vi "Autonomous Independent.vi"() -> ()   [LabVIEW 2014]
doc: "This VI is called when autonomous begins, and will automatically be terminated when autonomous ends. You can carry out timed or sensor driven robot movement independently without needing to return to the caller."
uses:
  Auto/Autonomous Modes.ctl
  Elevator/Elevator States.ctl
  Arms/Arm clapper state.ctl
  Utilities/Sensor Refname.ctl
  Utilities/Sensor Refname to String.vi
  <vilib>/Rock Robotics/Network Tables/SD Read Number.vi
panel:
  in  "Turn gyro":T1={"proportional gain (Kc)"=-0.05625, "integral time (Ti, min)"=0.0, "derivative time (Td, min)"=0.0} {"derivative time (Td, min)" format="%.3f"; "integral time (Ti, min)" format="%.3f"; "proportional gain (Kc)" format="%.3f"}
  in  "Third Forward Speed":dbl=0.7
  in  "Deposit Stack Drive Speed":dbl=-0.8 format="%#_13g"
  in  "Forward Speed Second Movement":dbl=0.65
  in  "Forward Speed into Zone":dbl=-0.8
  in  "Forward Speed First":dbl=0.8 format="%#_13g"
  in  "Distance (in)":dbl=57.0
  in  "Turn Left Distance (in)":dbl=90.0 format="%#_13g"
  in  "Turn Left Speed":dbl=0.75
  in  "Turn Right Speed":dbl=0.75
  in  "Turn Right Distance (in)":dbl=90.0 format="%#_13g"
  in  "Move Speed":dbl=0.75 format="%#_13g"
  in  "Move Time (s)":dbl=2.5 format="%#_13g"
  # "THREE TOTE"
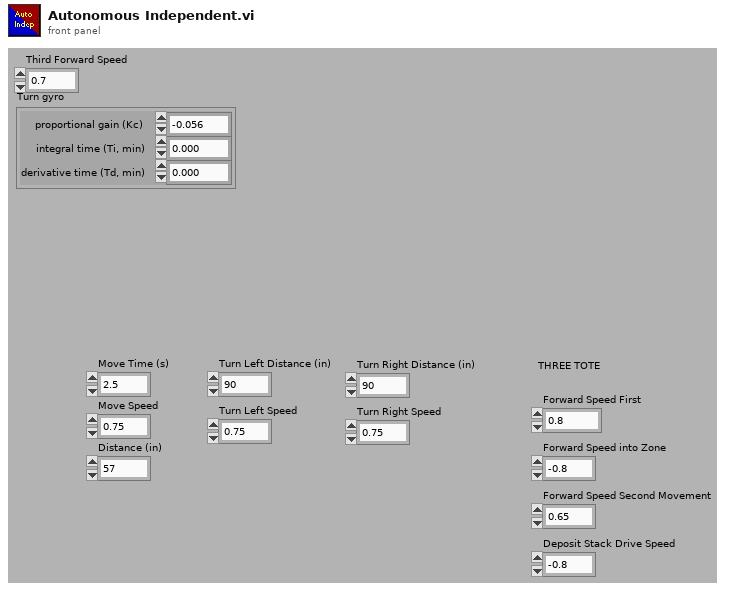
[diagram p1: front panel]
types:
  T1 = cluster{"proportional gain (Kc)":dbl, "integral time (Ti, min)":dbl, "derivative time (Td, min)":dbl}
  T2 = typedef "Autonomous Modes.ctl" = enum16{"3 Tote", "Turn Left, Drive to Auto", "Turn Right, Drive to Auto", "1 Bin", "Move To Auto Zone", "Do Nothing"}
  T3 = typedef "Auto Notifiers.ctl" = cluster{"Auto to Clap":refnum<notifier>, "Clap to Auto":refnum<notifier>, "Auto to Angle":refnum<notifier>, "Angle to Auto":refnum<notifier>, "Auto to Roller":refnum<notifier>, "Drive Distance Speed":refnum<notifier>, "Drive Distance Distance":refnum<notifier>, "Auto Done?":refnum<notifier>, "Keep Straight?":refnum<notifier>, "Turn 90?":refnum<notifier>}
  T4 = typedef "Auto Refs.ctl" = cluster{"Ultrasonic Forward":T5, "Ultrasonic Back":T5, "Strafe Motor":T9, "Drive Motors":T18, "Gyro":T19}
  T5 = typedef "WPI_SonarMB1010AnalogDeviceRef.ctl" = cluster{"AIDeviceRef":T6, "Scaling factor (V/in)":dbl, "Average Bits":u8}
  T6 = typedef "WPI_AnalogChannelDevRef.ctl" = cluster{"DevStatus":errorcluster, "Controller":T7, "Analog Channel":T8}
  T7 = typedef "FPGA_TypedefAnalogModule.ctl" = enum16{"Controller 1"}
  T8 = typedef "FPGA_AIChannel.ctl" = enum8{"AI 0", "AI 1", "AI 2", "AI 3", "AI MXP 0", "AI MXP 1", "AI MXP 2", "AI MXP 3", "Invalid"}
  T9 = typedef "WPI_MotorControlDeviceRef.ctl" = cluster{"DeviceStatus":errorcluster, "Type":T10, "PWM":cluster{"Controller":T11, "PWM Channel":T12, "DeadBand":T13}, "CAN":cluster{"Device Number":u8, "Control Mode":T14, "Semaphore":T15, "Max Vout":dbl, "TalonSRX Control Mode":T16}, "Invert":bool, "TransformRef":T17, "InvTransformRef":T17}
  T10 = typedef "WPI_MotorControlType.ctl" = enum16{"PWM", "CAN", "CANTalonSRX"}
  T11 = typedef "FPGA_TypedefDigitalModule.ctl" = enum16{"Controller 1"}
  T12 = typedef "FPGA_DIOPWMChannel.ctl" = enum8{"PWM 0", "PWM 1", "PWM 2", "PWM 3", "PWM 4", "PWM 5", "PWM 6", "PWM 7", "PWM 8", "PWM 9", "PWM MXP 0", "PWM MXP 1", "PWM MXP 2", "PWM MXP 3", "PWM MXP 4", "PWM MXP 5", "PWM MXP 6", "PWM MXP 7", "PWM MXP 8", "PWM MXP 9", "Invalid"}
  T13 = typedef "WPI_PWMDeadband.ctl" = cluster{"Name":string, "maxPositivePwm":i32, "minPositivePwm":i32, "centerPwm":i32, "maxNegativePwm":i32, "minNegativePwm":i32, "angularRange":u16}
  T14 = typedef "WPI_CANJaguar_ControlMode.ctl" = enum8{"Percent VBus", "Current", "Speed", "Position", "Voltage"}
  T15 = typedef "Semaphore RefNum" = refnum<k1>
  T16 = typedef "WPI_CANTalonSRX_APIControlMode.ctl" = enum8{"Percent VBus", "Speed", "Position", "Slave", "Unchanged / Invalid"}
  T17 = typedef "WPI_PWMTransform_ConPane.ctl" = refnum<vi>
  T18 = typedef "WPI_RobotDriveDevRef.ctl" = cluster{"DevStatus":errorcluster, "Motors[]":T9[], "Square Inputs":bool, "Max Output":dbl}
  T19 = typedef "WPI_GyroDevRef.ctl" = cluster{"DevStatus":errorcluster, "Analog Module":T7, "Analog Channel":T8, "Offset":dbl, "Gain (VoltsPerDegree/Second)":dbl}
  T20 = typedef "Sensor Refname.ctl" = enum16{"Gyro", "Elevator Top LS", "Elevator Bottom LS", "Claw Outside LS", "Left Drive Encoder", "Right Drive Encoder", "Strafe Encoder", "Elevator Encoder", "Ultrasonic Forward", "Ultrasonic Back", "Arm Angle POT", "Arm Clapper POT", "Accelerometer", "Tote LS", "DIP 1", "DIP 2", "DIP 3", "DIP 4"}
  T21 = typedef "Arm clapper state.ctl" = enum16{"In", "Tote Closed", "Bin Closed", "Straight", "Open"}
  T22 = typedef "Elevator States.ctl" = enum16{"Ground", "Tote 1", "Tote 2", "Tote 3", "Tote 4", "Tote 5", "Tote 6"}
  T23 = typedef "WPI_SwitchDevRef.ctl" = cluster{"DevStatus":errorcluster, "DIO Channel":T24, "Controller":T11, "CntIndex":T25, "Normally Closed":bool}
  T24 = typedef "FPGA_DIOChannel.ctl" = enum8{"DIO 0", "DIO 1", "DIO 2", "DIO 3", "DIO 4", "DIO 5", "DIO 6", "DIO 7", "DIO 8", "DIO 9", "DIO MXP 0", "DIO MXP 1", "DIO MXP 2", "DIO MXP 3", "DIO MXP 4", "DIO MXP 5", "DIO MXP 6", "DIO MXP 7", "DIO MXP 8", "DIO MXP 9", "DIO MXP 10", "DIO MXP 11", "DIO MXP 12", "DIO MXP 13", "DIO MXP 14", "DIO MXP 15", "Invalid"}
  T25 = typedef "FPGA_CounterCtrSystemIndex.ctl" = enum8{"Ctr 0", "Ctr 1", "Ctr 2", "Ctr 3", "Ctr 4", "Ctr 5", "Ctr 6", "Ctr 7", "Invalid"}
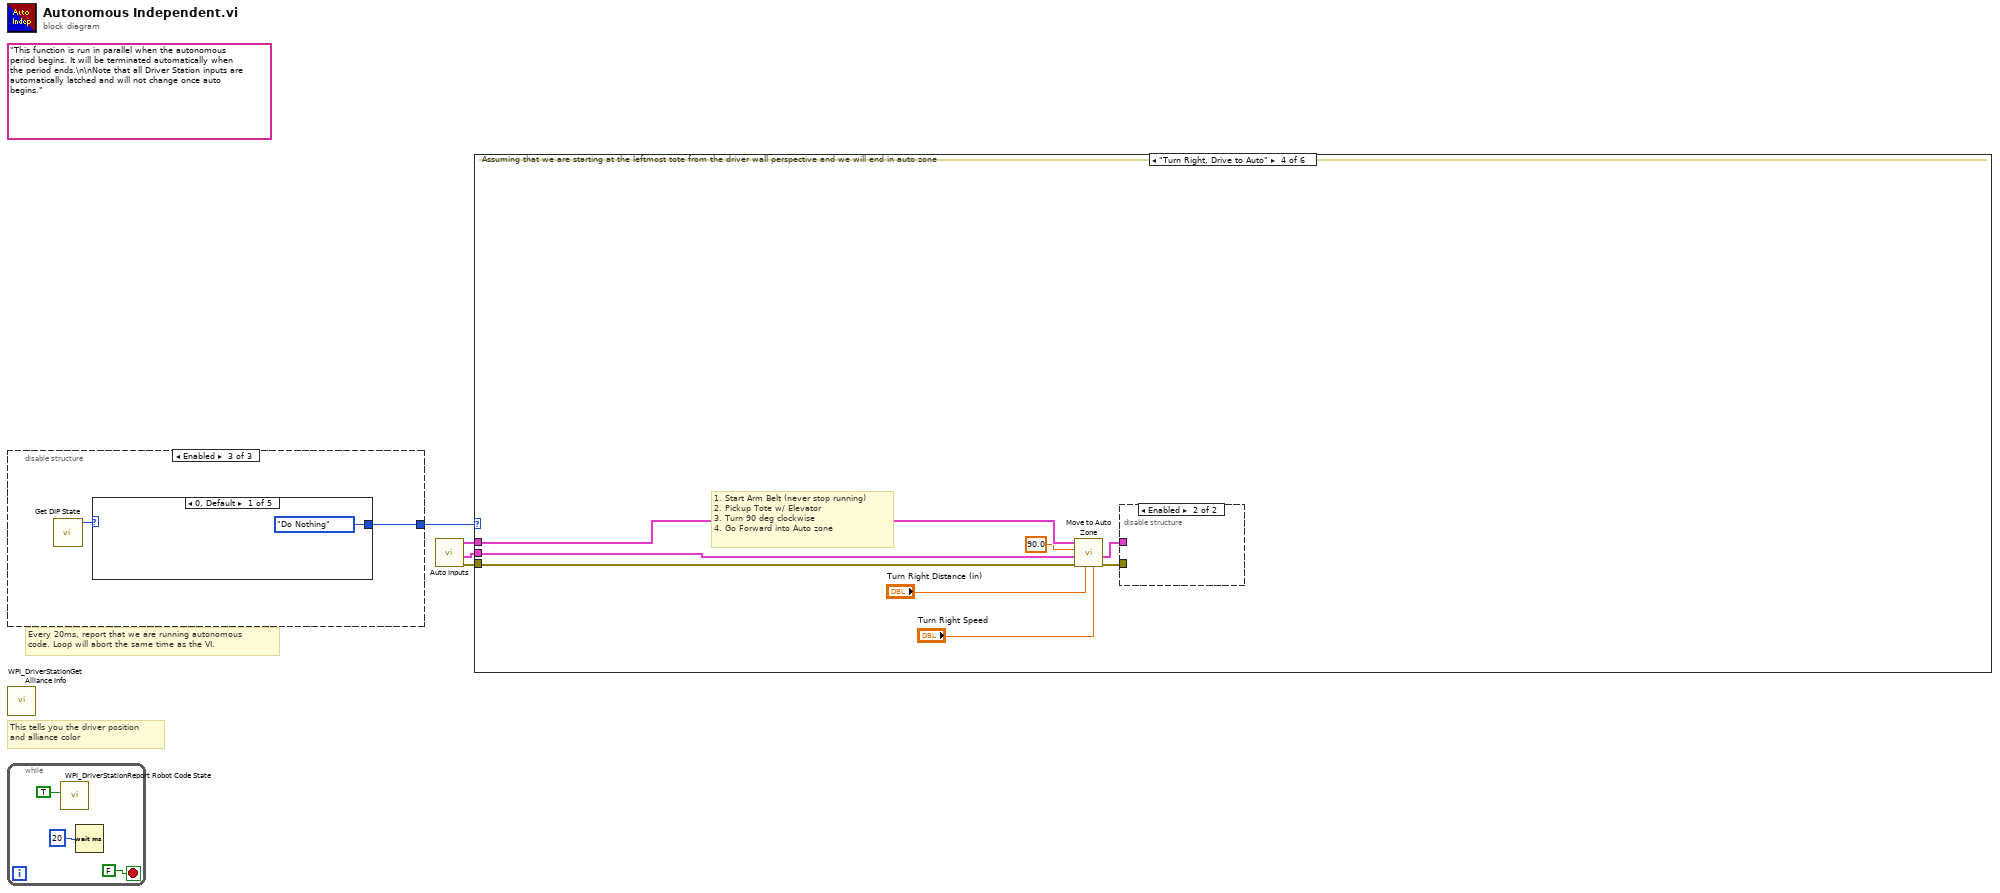
[diagram p0: block diagram]
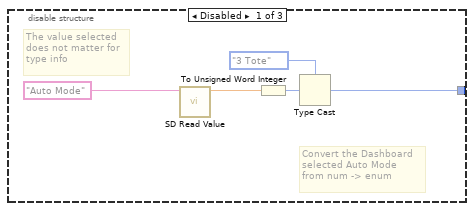
[diagram p2: hidden frame]
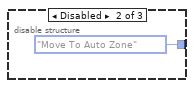
[diagram p3: hidden frame]
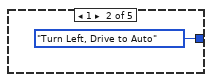
[diagram p4: hidden frame]
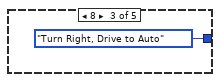
[diagram p5: hidden frame]
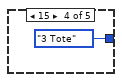
[diagram p6: hidden frame]
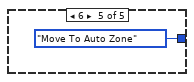
[diagram p7: hidden frame]
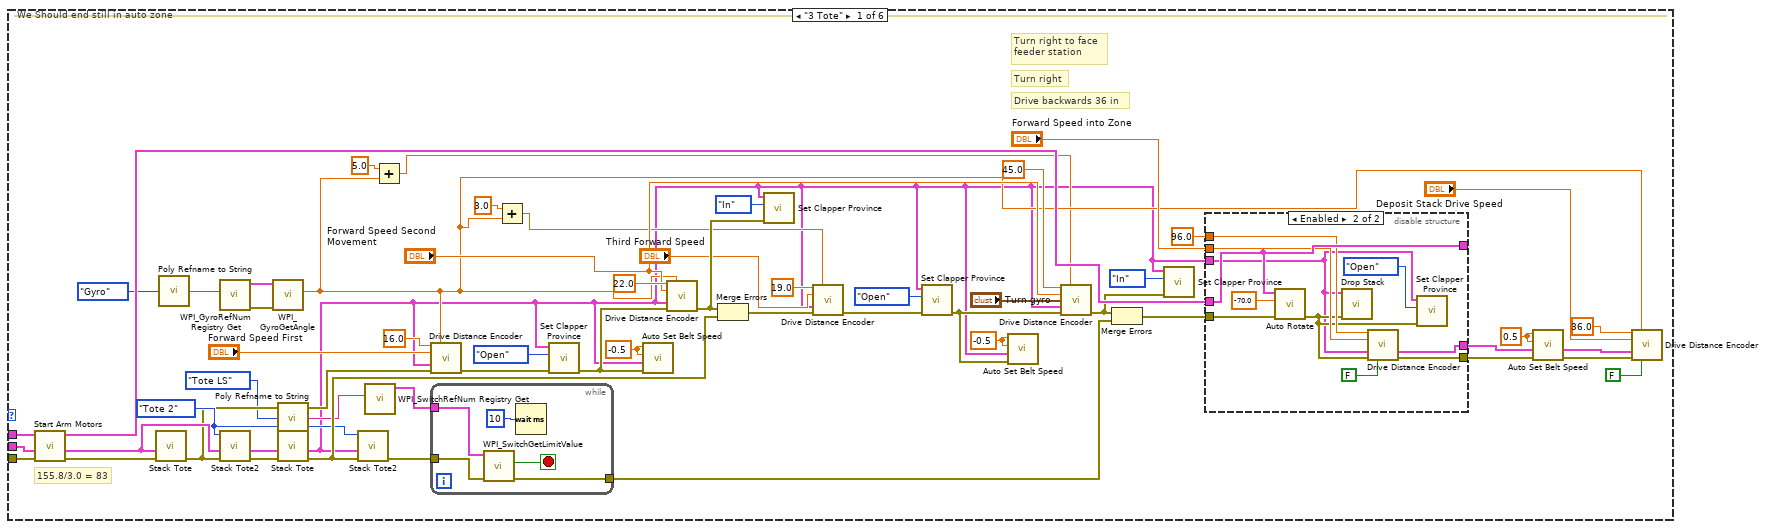
[diagram p8: hidden frame]
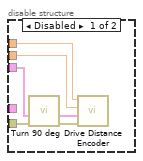
[diagram p9: hidden frame]
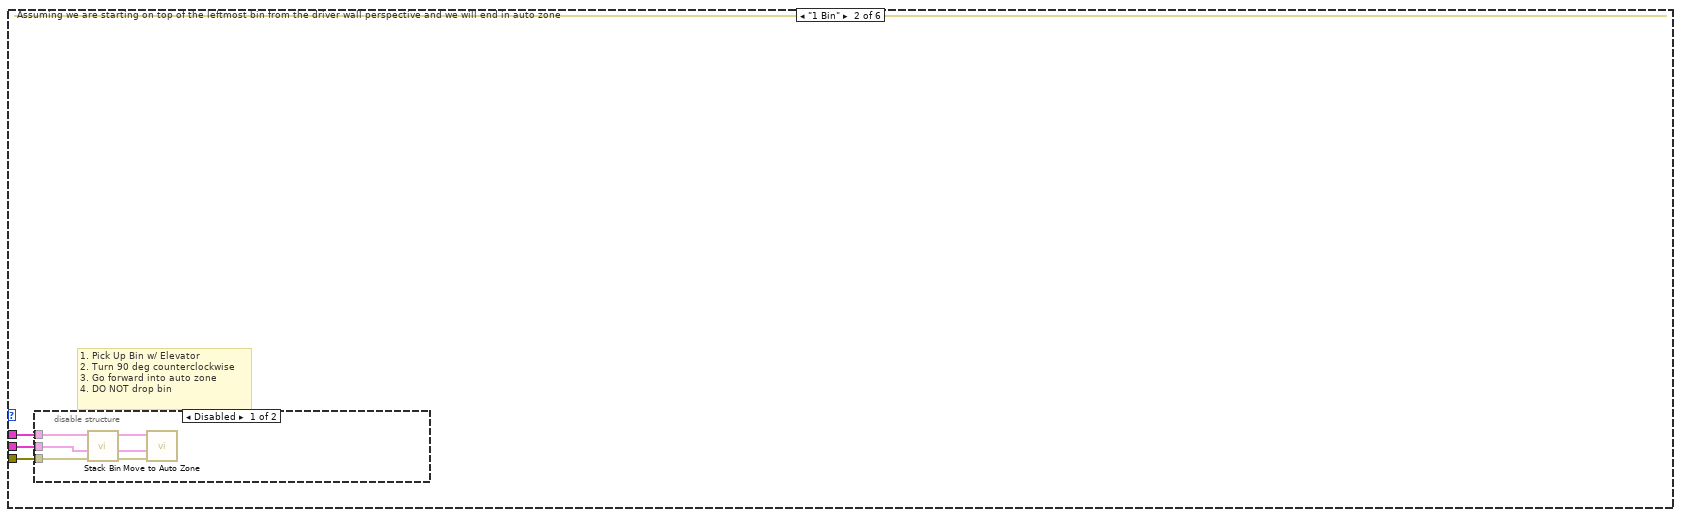
[diagram p10: hidden frame]
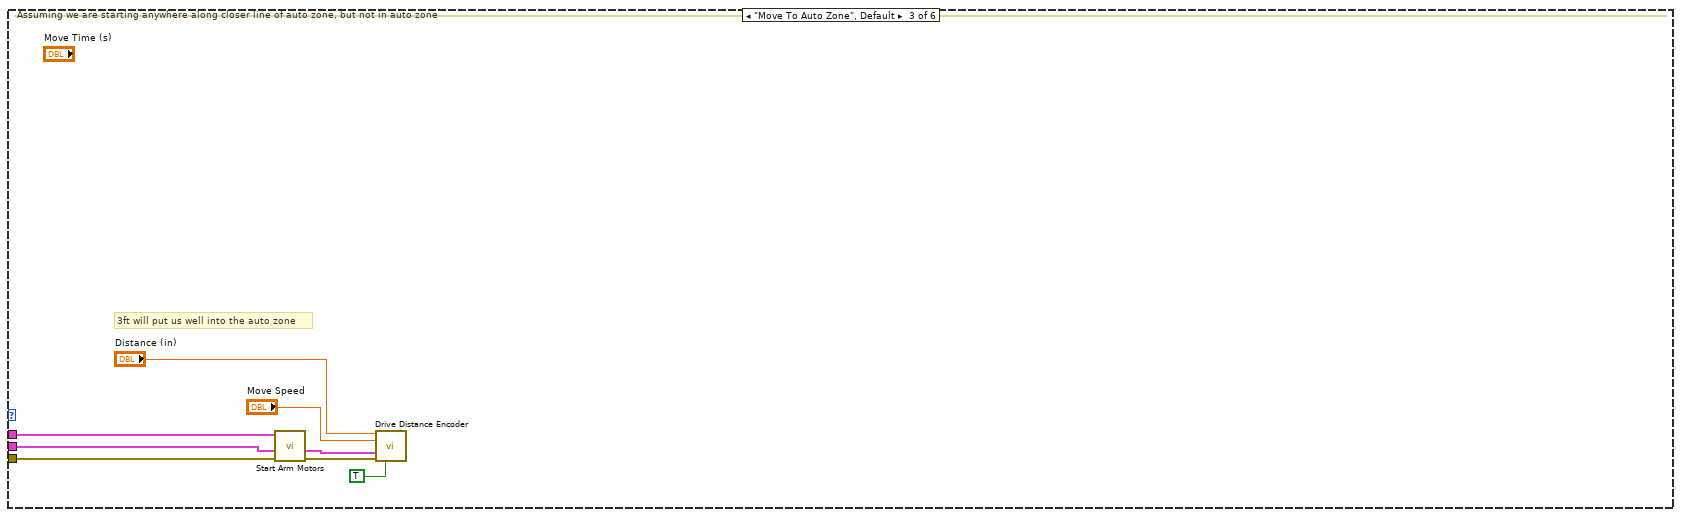
[diagram p12: hidden frame]
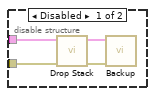
[diagram p13: hidden frame]
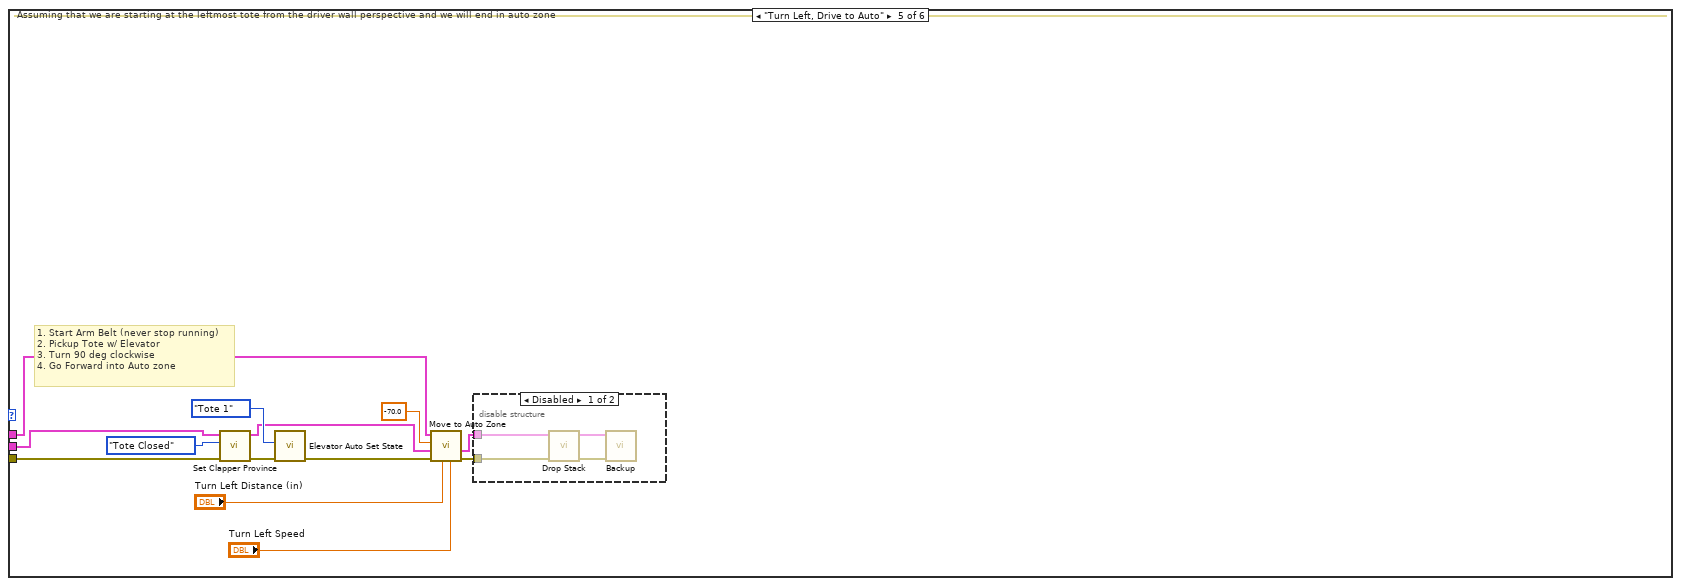
[diagram p14: hidden frame]
diagram:
  (unwired) "This function is run in parallel when the autonomous period begins. It will be terminated automatically when the period ends.\n\nNote that all Driver Station inputs are automatically latched and will not change once auto begins."
  # "Every 20ms, report that we are running autonomous\ncode. Loop will abort the same time as the VI."
  # "This tells you the driver position\nand alliance color"
  n1 = disable-structure shown="Enabled" {
    disable-tunnel: [w5 Autonomous_Modes."Move To Auto Zone" ("Auto Mode") w11] -> w1
    frame Disabled {
      # "The value selected\ndoes not matter for\ntype info"
      # "Convert the Dashboard\nselected Auto Mode\nfrom num -> enum"
      n2 = call-poly <vilib>:"SD Read Value.vi"("Name"="Auto Mode") -> ("Numeric"=w9:dbl)  [unwired: 8 in, 2 out]
      n3 = To Unsigned Word Integer(number=w9) -> (unsigned 16bit integer=w8:u16)
      n4 = Type Cast(type=Autonomous_Modes."3 Tote" ("Auto Mode"), x=w8) -> (*(type *) &x=w5:T2)
    }
    frame Disabled {
    }
    frame Enabled {
      n5 = call "Get DIP State.vi"() -> ("DIP State"=w12:u32)  [unwired: 10 in, 1 out]
      n6 = case shown="0, Default" w12 {
        tunnel: [Autonomous_Modes."Do Nothing" ("Auto Mode") Autonomous_Modes."Turn Left, Drive to Auto" ("Auto Mode") Autonomous_Modes."Turn Right, Drive to Auto" ("Auto Mode") Autonomous_Modes."3 Tote" ("Auto Mode") Autonomous_Modes."Move To Auto Zone" ("Auto Mode")] -> w11
        frame 0, Default {
        }
        frame 1 {
        }
        frame 8 {
        }
        frame 15 {
        }
        frame 6 {
        }
      }
    }
  }
  n7 = call <vilib>:"WPI_DriverStationGet Alliance Info.vi"() -> ()  [unwired: 12 out]
  n8 = while {
    stop <- FALSE stop-if-true
    n9 = call <vilib>:"WPI_DriverStationReport Robot Code State.vi"("Autonomous"=TRUE) -> ()  [unwired: 10 in, 1 out]
    n10 = Wait (ms)(milliseconds to wait=u32 20) -> ()  [unwired: 1 out]
  }
  n11 = call "Auto Inputs.vi"() -> ("error out"=w2:errorcluster, "Auto Notifiers Out"=w3:T3, "Auto Refs"=w4:T4)  [unwired: 9 in]
  n12 = case shown="\"Turn Right, Drive to Auto\"" w1 {
    tunnel: w4 -> [w76 w103 w112 w121 w139 _]
    tunnel: w3 -> [w78 w102 w114 w123 w133 _]
    tunnel: w2 -> [w77 w101 w116 w124 w141 _]
    frame "3 Tote" {
      w57 = -0.5 ("Right Belt")
      w68 = -0.5 ("Right Belt")
      w42 = Elevator_States."Tote 2" ("New State")
      w72 = 0.5
      # "Drive backwards 36 in"
      # "Turn right to face\nfeeder station"
      # "Turn right"
      # "155.8/3.0 = 83"
      # "We Should end still in auto zone"
      n13 = call "Start Arm Motors.vi"("error in"=w77, "Auto Notifiers In"=w78, "Auto Refs"=w76) -> ("error out"=w47:errorcluster, "Auto Notifiers Out"=w41:T3, "Auto Refs"=w74:T4)  [unwired: 6 in]
      n14 = call "Stack Tote.vi"("error in"=w47, "Auto Notifiers In"=w41) -> ("error out(no error)"=w38:errorcluster)  [unwired: 8 in, 1 out]
      n15 = call-poly "Poly Refname to String.vi"("Sensor Refnames"=Sensor_Refname."Gyro") -> ("Refname"=w49:string)
      n16 = call <vilib>:"WPI_GyroRefNum Registry Get.vi"("refnum name"=w49) -> ("error out"=w48:errorcluster, "GyroDevRef"=w51:T19)  [unwired: 9 in]
      n17 = call "Stack Tote2.vi"("error in (no error)"=w38, "Auto Notifiers In"=w41, "End at"=w42) -> ("error out"=w39:errorcluster, "Auto Notifiers Out"=w22:T3)  [unwired: 7 in]
      n18 = call <vilib>:"WPI_GyroGetAngle.vi"("error in (no error)"=w48, "GyroDevRef"=w51) -> ("Angle"=w36:dbl)  [unwired: 6 in, 3 out]
      n19 = call-poly "Poly Refname to String.vi"("Sensor Refnames"=Sensor_Refname."Tote LS") -> ("Refname"=w31:string)
      n20 = call "Stack Tote.vi"("error in"=w39, "Auto Notifiers In"=w22) -> ("error out(no error)"=w43:errorcluster, "Auto Notifiers Out"=w21:T3)  [unwired: 8 in]
      n21 = call "Stack Tote2.vi"("error in (no error)"=w43, "Auto Notifiers In"=w21, "End at"=w42) -> ("error out"=w30:errorcluster)  [unwired: 7 in, 1 out]
      n22 = call <vilib>:"WPI_SwitchRefNum Registry Get.vi"("refnum name"=w31) -> ("SwitchDevRef"=w32:T23)  [unwired: 9 in, 1 out]
      n23 = Add(x=5.0 ("y"), y=w36) -> (x+y=w35:dbl)
      n24 = call "Drive Distance Encoder.vi"("Distance (in)"=16.0, "Gyro setpoint"=w36, "Speed"="Forward Speed First", "Auto Notifiers In"=w21, "error in"=w38) -> ("error out"=w64:errorcluster)  [unwired: 9 in, 1 out]
      n25 = while {
        tunnel: w30 -> [w80]
        tunnel: [w81] -> w29
        tunnel: w32 -> [w82]
        stop <- w83 stop-if-true
        n26 = call <vilib>:"WPI_SwitchGetLimitValue.vi"("error in (no error)"=w80, "SwitchDevRef"=w82) -> ("error out"=w81:errorcluster, "Switch Pressed"=w83:bool)  [unwired: 7 in, 1 out]
        n27 = Wait (ms)(milliseconds to wait=u32 10) -> ()  [unwired: 1 out]
      }
      n28 = Add(x=3.0, y=w36) -> (x+y=w24:dbl)
      n29 = call "Set Clapper Province.vi"("error in"=w64, "Enum"=Arm_clapper_state."Open", "Auto Notifiers In"=w21) -> ("error out"=w63:errorcluster)  [unwired: 7 in, 1 out]
      n30 = call "Auto Set Belt Speed.vi"("error in"=w63, "Auto Notifiers In"=w21, "Right Belt"=w68, "Left Belt"=w68) -> ()  [unwired: 6 in, 2 out]
      n31 = call "Drive Distance Encoder.vi"("Distance (in)"=22.0, "Gyro setpoint"=w36, "Speed"="Forward Speed Second Movement", "Auto Notifiers In"=w21, "error in"=w63) -> ("error out"=w45:errorcluster)  [unwired: 9 in, 1 out]
      n32 = Merge Errors(w45, w43) -> (w55:errorcluster)
      n33 = call "Set Clapper Province.vi"("error in"=w45, "Enum"=Arm_clapper_state."In", "Auto Notifiers In"=w21) -> ()  [unwired: 7 in, 2 out]
      n34 = call "Drive Distance Encoder.vi"("Distance (in)"=19.0, "Gyro setpoint"=w24, "Speed"="Third Forward Speed", "Auto Notifiers In"=w21, "error in"=w55) -> ("error out"=w61:errorcluster)  [unwired: 9 in, 1 out]
      n35 = call "Set Clapper Province.vi"("error in"=w61, "Enum"=Arm_clapper_state."Open", "Auto Notifiers In"=w21) -> ("error out"=w62:errorcluster)  [unwired: 7 in, 1 out]
      n36 = call "Auto Set Belt Speed.vi"("error in"=w62, "Auto Notifiers In"=w21, "Right Belt"=w57, "Left Belt"=w57) -> ()  [unwired: 6 in, 2 out]
      n37 = call "Drive Distance Encoder.vi"("Distance (in)"=45.0, "Gyro setpoint"=w35, "Speed"="Forward Speed Second Movement", "Gyro gains"="Turn gyro", "Auto Notifiers In"=w21, "error in"=w62) -> ("error out"=w44:errorcluster)  [unwired: 8 in, 1 out]
      n38 = Merge Errors(w44, w29) -> (w53:errorcluster)
      n39 = call "Set Clapper Province.vi"("error in"=w44, "Enum"=Arm_clapper_state."In", "Auto Notifiers In"=w21) -> ()  [unwired: 7 in, 2 out]
      n40 = disable-structure shown="Enabled" {
        disable-tunnel: w53 -> [w89 w98]
        disable-tunnel: w21 -> [w88 w90]
        disable-tunnel: "Forward Speed into Zone" -> [w85 w95]
        disable-tunnel: 96.0 ("Distance (in)") -> [w84 w96]
        disable-tunnel: w74 -> [_ w100]
        disable-tunnel: [_ w100] -> _
        disable-tunnel: [_ w93] -> w28
        disable-tunnel: [_ w92] -> w27
        frame Disabled {
          n41 = call "Turn 90 deg.vi"("error in"=w89, "Auto Notifiers In"=w88) -> ("error out"=w87:errorcluster, "Auto Notifiers Out"=w86:T3)  [unwired: 8 in]
          n42 = call "Drive Distance Encoder.vi"("error in"=w87, "Auto Notifiers In"=w86, "Speed"=w85, "Distance (in)"=w84) -> ()  [unwired: 6 in, 2 out]
        }
        frame Enabled {
          n43 = call "Auto Rotate.vi"("error in (no error)"=w98, "Rotation"=-70.0 ("Rotation (deg)"), "Auto Refs"=w100) -> ("error out"=w91:errorcluster)  [unwired: 8 in]
          n44 = call "Drop Stack.vi"("error in"=w91, "Auto Notifiers In"=w90) -> ()  [unwired: 8 in, 2 out]
          n45 = call "Drive Distance Encoder.vi"("Distance (in)"=w96, "Speed"=w95, "Auto Notifiers In"=w90, "error in"=w91, "Gyro Sync?"=FALSE) -> ("Auto Notifiers Out"=w92:T3, "error out"=w93:errorcluster)  [unwired: 9 in]
          n46 = call "Set Clapper Province.vi"("error in"=w91, "Enum"=Arm_clapper_state."Open", "Auto Notifiers In"=w90) -> ()  [unwired: 7 in, 2 out]
        }
      }
      n47 = call "Auto Set Belt Speed.vi"("error in"=w28, "Auto Notifiers In"=w27, "Right Belt"=w72, "Left Belt"=w72) -> ("error out"=w26:errorcluster, "Auto Notifiers Out"=w25:T3)  [unwired: 6 in]
      n48 = call "Drive Distance Encoder.vi"("Distance (in)"=36.0, "Gyro setpoint"=w36, "Speed"="Deposit Stack Drive Speed", "Auto Notifiers In"=w25, "error in"=w26, "Gyro Sync?"=FALSE) -> ()  [unwired: 8 in, 2 out]
    }
    frame "1 Bin" {
      # "1. Pick Up Bin w/ Elevator\n2. Turn 90 deg counterclockwise\n3. Go forward into auto zone\n4. DO NOT drop bin"
      # "Assuming we are starting on top of the leftmost bin from the driver wall perspective and we will end in auto zone"
      n49 = disable-structure shown="Disabled" {
        disable-tunnel: w103 -> [w107 _]
        disable-tunnel: w102 -> [w106 _]
        disable-tunnel: w101 -> [w104 _]
        frame Disabled {
          n50 = call "Stack Bin.vi"("error in"=w104, "Auto Notifiers In"=w106, "Auto Refs"=w107) -> ("error out"=w109:errorcluster, "Auto Notifiers Out"=w105:T3, "Auto Refs"=w108:T4)  [unwired: 6 in]
          n51 = call "Move to Auto Zone.vi"("error in"=w109, "Auto Notifiers In"=w105, "Auto Refs"=w108) -> ()  [unwired: 7 in, 2 out]
        }
        frame Enabled {
        }
      }
    }
    frame "Move To Auto Zone", Default {
      # "3ft will put us well into the auto zone"
      # "Assuming we are starting anywhere along closer line of auto zone, but not in auto zone"
      n52 = call "Start Arm Motors.vi"("error in"=w116, "Auto Notifiers In"=w114, "Auto Refs"=w112) -> ("error out"=w115:errorcluster, "Auto Notifiers Out"=w113:T3)  [unwired: 6 in, 1 out]
      n53 = call "Drive Distance Encoder.vi"("Distance (in)"="Distance (in)", "Speed"="Move Speed", "Auto Notifiers In"=w113, "error in"=w115, "Gyro Sync?"=TRUE) -> ()  [unwired: 9 in, 2 out]
    }
    frame "Turn Right, Drive to Auto" {
      # "1. Start Arm Belt (never stop running)\n2. Pickup Tote w/ Elevator\n3. Turn 90 deg clockwise\n4. Go Forward into Auto zone"
      # "Assuming that we are starting at the leftmost tote from the driver wall perspective and we will end in auto zone"
      n54 = call "Move to Auto Zone.vi"("Speed"="Turn Right Speed", "Distance (m)"="Turn Right Distance (in)", "error in"=w124, "Auto Notifiers In"=w123, "Rotation (deg)"=90.0, "Auto Refs"=w121) -> ("error out"=w125:errorcluster, "Auto Notifiers Out"=w122:T3)  [unwired: 4 in]
      n55 = disable-structure shown="Enabled" {
        disable-tunnel: w125 -> [w128 _]
        disable-tunnel: w122 -> [w127 _]
        frame Disabled {
          n56 = call "Drop Stack.vi"("error in"=w128, "Auto Notifiers In"=w127) -> ("error out"=w129:errorcluster, "Auto Notifiers Out"=w126:T3)  [unwired: 8 in]
          n57 = call "Backup.vi"("error in"=w129, "Auto Notifiers In"=w126) -> ()  [unwired: 8 in, 2 out]
        }
        frame Enabled {
        }
      }
    }
    frame "Turn Left, Drive to Auto" {
      # "1. Start Arm Belt (never stop running)\n2. Pickup Tote w/ Elevator\n3. Turn 90 deg clockwise\n4. Go Forward into Auto zone"
      # "Assuming that we are starting at the leftmost tote from the driver wall perspective and we will end in auto zone"
      n58 = call "Set Clapper Province.vi"("error in"=w141, "Enum"=Arm_clapper_state."Tote Closed", "Auto Notifiers In"=w133) -> ("error out"=w131:errorcluster, "Auto Notifiers Out"=w130:T3)  [unwired: 7 in]
      n59 = call "Elevator Auto Set State.vi"("error in (no error)"=w131, "New State"=Elevator_States."Tote 1") -> ("error out"=w135:errorcluster)  [unwired: 9 in]
      n60 = call "Move to Auto Zone.vi"("Speed"="Turn Left Speed", "Distance (m)"="Turn Left Distance (in)", "error in"=w135, "Auto Notifiers In"=w130, "Rotation (deg)"=-70.0, "Auto Refs"=w139) -> ("error out"=w142:errorcluster, "Auto Notifiers Out"=w140:T3)  [unwired: 4 in]
      n61 = disable-structure shown="Disabled" {
        disable-tunnel: w142 -> [w145 _]
        disable-tunnel: w140 -> [w144 _]
        frame Disabled {
          n62 = call "Drop Stack.vi"("error in"=w145, "Auto Notifiers In"=w144) -> ("error out"=w146:errorcluster, "Auto Notifiers Out"=w143:T3)  [unwired: 8 in]
          n63 = call "Backup.vi"("error in"=w146, "Auto Notifiers In"=w143) -> ()  [unwired: 8 in, 2 out]
        }
        frame Enabled {
        }
      }
    }
    frame "Do Nothing" {
    }
  }
